vi "NHMFL SCMPS Init Sw Heater.vi"() -> (0 "Persistent Field":dbl=1.0 format="%.2f")   [LabVIEW 2025]
doc: "Author: Scott Hannahs <sth@magnet.fsu.edu>\n\nThis software is licensed for use under the “MIT License\"\nCopyright (c) 2025 Scott Hannahs, sth@sth@magnet.sthnet.net\n\nPermission is hereby granted, free of charge, to any person obtaining a copy of this software and associated documentation files (the \"Software\"), to deal in the Software without restriction, including without limitation the rights to use, copy, modify, merge, publish, distribute, sublicense, and/or sell copies of the Software, and to permit persons to whom the Software is furnished to do so, subject to the following conditions: The above copyright notice and this permission notice shall be included in all copies or substantial portions of the Software.\n\nTHE SOFTWARE IS PROVIDED \"AS IS\", WITHOUT WARRANTY OF ANY KIND, EXPRESS OR IMPLIED, INCLUDING BUT NOT LIMITED TO THE WARRANTIES OF MERCHANTABILITY, FITNESS FOR A PARTICULAR PURPOSE AND NONINFRINGEMENT. IN NO EVENT SHALL THE AUTHORS OR COPYRIGHT HOLDERS BE LIABLE FOR ANY CLAIM, DAMAGES OR OTHER LIABILITY, WHETHER IN AN ACTION OF CONTRACT, TORT OR OTHERWISE, ARISING FROM, OUT OF OR IN CONNECTION WITH THE SOFTWARE OR THE USE OR OTHER DEALINGS IN THE SOFTWARE."
panel:
  in  "OK Button":bool
  in  "Magnet Field":dbl format="%.2f"
  # "The switch heater is off!\nPlease enter the field in the magnet and hit ok.\nIf you do not know or are not sure \nget help from a mK staff member."
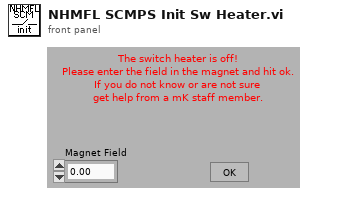
[diagram p1: front panel]
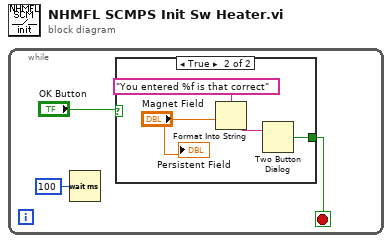
[diagram p0: block diagram]
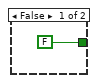
[diagram p2: hidden frame]
diagram:
  n1 = while {
    stop <- w2 stop-if-true
    n2 = Wait (ms)(milliseconds to wait=u32 100) -> ()  [unwired: 1 out]
    n3 = case shown="True" "OK Button" {
      tunnel: [FALSE w6] -> w2
      frame False {
      }
      frame True {
        n4 = Format Into String(format string="You entered %f is that correct", "Magnet Field") -> (resulting string=w8:string)  [unwired: 2 in, 1 out]
        n5 = Two Button Dialog(message=w8) -> (T button?=w6:bool)  [unwired: 2 in]
        "Persistent Field" <- "Magnet Field"
      }
    }
  }
